vi "Verileri GUI'ye Gönder_Harmonik.vi"(4 "Uygulanan Değerler":dbl[][](array[numeric]), 5 "GKÇ-1 FD2 Ic Değerleri":dbl[][](array[numeric]), 6 "GKÇ-1 FD2 Ib Değerleri":dbl[][](array[numeric]), 7 "GKÇ-1 FD2 Ia Değerleri":dbl[][](array[numeric]), 8 "GKÇ-1 FD1 Ic Değerleri":dbl[][](array[numeric]), 9 "GKÇ-1 FD1 Ib Değerleri":dbl[][](array[numeric]), 10 "GKÇ-1 FD1 Ia Değerleri":dbl[][](array[numeric]), 11 "GKÇ-1 Akım Harmonik_Limit_Değerleri":dbl[][](array[numeric])) -> ()   [LabVIEW 2014]
uses:
  VeriPaylasim_Globali.vi
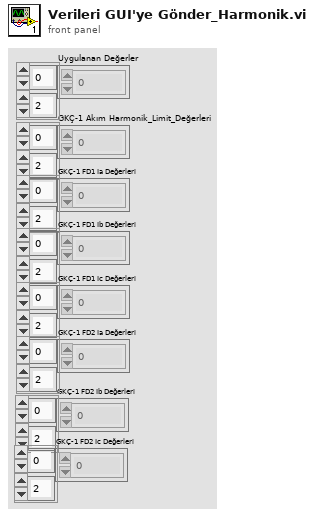
[diagram p1: front panel]
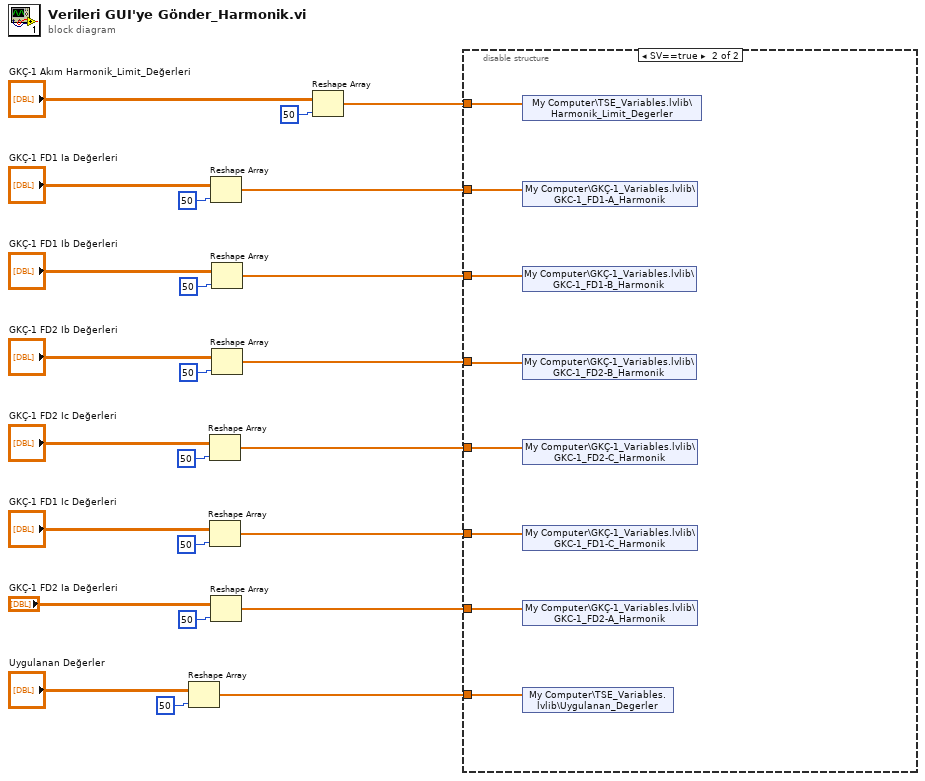
[diagram p0: block diagram]
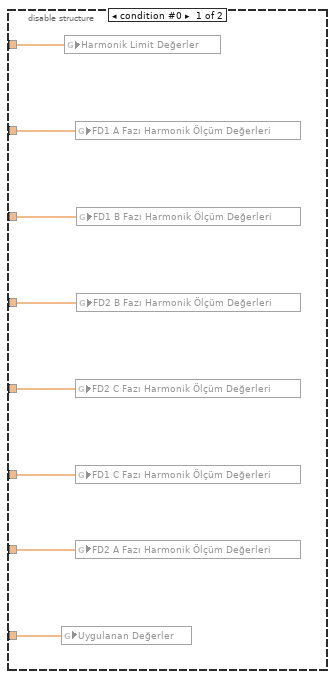
[diagram p2: hidden frame]
diagram:
  n1 = Reshape Array("Uygulanan Değerler", 50 ("dimension size")) -> (w8:dbl[])
  n2 = Reshape Array("GKÇ-1 FD2 Ic Değerleri", 50 ("dimension size")) -> (w3:dbl[])
  n3 = Reshape Array("GKÇ-1 FD1 Ic Değerleri", 50 ("dimension size")) -> (w2:dbl[])
  n4 = Reshape Array("GKÇ-1 FD1 Ia Değerleri", 50 ("dimension size")) -> (w6:dbl[])
  n5 = Reshape Array("GKÇ-1 FD2 Ia Değerleri", 50 ("dimension size")) -> (w1:dbl[])
  n6 = Reshape Array("GKÇ-1 FD1 Ib Değerleri", 50 ("dimension size")) -> (w5:dbl[])
  n7 = Reshape Array("GKÇ-1 FD2 Ib Değerleri", 50 ("dimension size")) -> (w4:dbl[])
  n8 = Reshape Array("GKÇ-1 Akım Harmonik_Limit_Değerleri", 50 ("dimension size")) -> (w7:dbl[])
  n9 = disable-structure shown="SV==true" {
    disable-tunnel: w8 -> [w32 w39]
    disable-tunnel: w7 -> [w31 w40]
    disable-tunnel: w6 -> [w30 w38]
    disable-tunnel: w5 -> [w29 w37]
    disable-tunnel: w4 -> [w28 w34]
    disable-tunnel: w3 -> [w27 w33]
    disable-tunnel: w2 -> [w26 w35]
    disable-tunnel: w1 -> [w25 w36]
    frame condition #0 {
      n10 = global write "VeriPaylasim_Globali.vi" "Uygulanan Değerler"(w32) -> ()
      n11 = global write "VeriPaylasim_Globali.vi" "Harmonik Limit Değerler"(w31) -> ()
      n12 = global write "VeriPaylasim_Globali.vi" "FD1 A Fazı Harmonik Ölçüm Değerleri"(w30) -> ()
      n13 = global write "VeriPaylasim_Globali.vi" "FD2 C Fazı Harmonik Ölçüm Değerleri"(w27) -> ()
      n14 = global write "VeriPaylasim_Globali.vi" "FD1 C Fazı Harmonik Ölçüm Değerleri"(w26) -> ()
      n15 = global write "VeriPaylasim_Globali.vi" "FD2 A Fazı Harmonik Ölçüm Değerleri"(w25) -> ()
      n16 = global write "VeriPaylasim_Globali.vi" "FD1 B Fazı Harmonik Ölçüm Değerleri"(w29) -> ()
      n17 = global write "VeriPaylasim_Globali.vi" "FD2 B Fazı Harmonik Ölçüm Değerleri"(w28) -> ()
    }
    frame condition #1 (active) {
      n18 = shared-variable "My Computer\\TSE_Variables.lvlib\\Harmonik_Limit_Degerler"(w40) -> ()  [unwired: 1 in, 1 out]
      n19 = shared-variable "My Computer\\GKÇ-1_Variables.lvlib\\GKC-1_FD1-A_Harmonik"(w38) -> ()  [unwired: 1 in, 1 out]
      n20 = shared-variable "My Computer\\GKÇ-1_Variables.lvlib\\GKC-1_FD1-B_Harmonik"(w37) -> ()  [unwired: 1 in, 1 out]
      n21 = shared-variable "My Computer\\GKÇ-1_Variables.lvlib\\GKC-1_FD2-B_Harmonik"(w34) -> ()  [unwired: 1 in, 1 out]
      n22 = shared-variable "My Computer\\GKÇ-1_Variables.lvlib\\GKC-1_FD2-C_Harmonik"(w33) -> ()  [unwired: 1 in, 1 out]
      n23 = shared-variable "My Computer\\GKÇ-1_Variables.lvlib\\GKC-1_FD1-C_Harmonik"(w35) -> ()  [unwired: 1 in, 1 out]
      n24 = shared-variable "My Computer\\GKÇ-1_Variables.lvlib\\GKC-1_FD2-A_Harmonik"(w36) -> ()  [unwired: 1 in, 1 out]
      n25 = shared-variable "My Computer\\TSE_Variables.lvlib\\Uygulanan_Degerler"(w39) -> ()  [unwired: 1 in, 1 out]
    }
  }
